vi "RevoxSerialTest.vi"() -> ()   [LabVIEW 2023]
uses:
  B203AllCluster.ctl
  B203Cluster.ctl
  <vilib>/Utility/error.llb/Trim Whitespace One-Sided.vi
  <instrlib>/_D2XX/D2XX/FT_Open_Device_By_Description.vi
  <instrlib>/_D2XX/D2XX-LV/private/FT_Status to Error.vi
  <instrlib>/_D2XX/D2XX-LV/API/Write Data (String).vi
  <instrlib>/_D2XX/D2XX-LV/API/Read Data (String).vi
  <instrlib>/_D2XX/D2XX-LV/D2XX-lv.lvlib
panel:
  out "String":string
  out "B203AllCluster":T1={"B203"={"Port"=enum."Anschluss 7", "Identifier"=0, "Language"=enum."Englisch", "Easy-Function"=enum."Easy Remote", "Timer-Function"=enum."Timer eingeschaltet", "Power ON condition"=enum."Lautsprecher A", "IR receiver"=enum."IR-Empfänger eingeschaltet"}, "Zeitstempel"=timestamp(0 s since 1904-01-01)} {"Zeitstempel" format="%<%x %.X>T"}
  in  "Stopp":bool
  in  "Schreibpuffer":string="0X"
  out "error out":errorcluster={"status"=FALSE, "code"=1073676294, "source"="VISA: Lesen in RevoxSerailTest.vi"} caption="Fehler (Ausgang)"
  in  "error in (no error)":errorcluster caption="Fehler (Eingang, kein Fehler)"
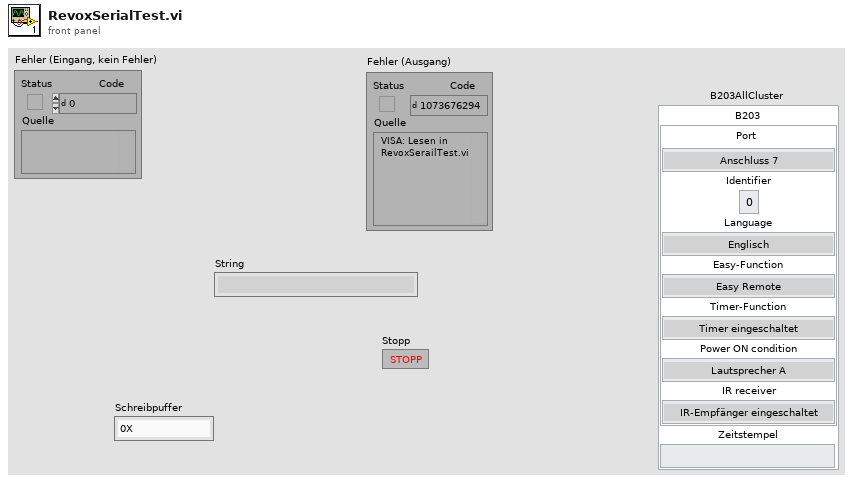
[diagram p1: front panel]
types:
  T1 = typedef "B203AllCluster.ctl" = cluster{"B203":T2, "Zeitstempel":timestamp}
  T2 = typedef "B203Cluster.ctl" = cluster{"Port":enum8{"B203-C", "Anschluss 1", "Anschluss 2", "Anschluss 3", "Anschluss 4", "Anschluss 5", "Anschluss 6", "Anschluss 7", "Anschluss 8", "Parallel Fernsteuerung"}, "Identifier":u8, "Language":enum8{"Englisch", "Deutsch", "Französich"}, "Easy-Function":enum8{"Easy Remote", "Easy Remote & Local", "Easy Off"}, "Timer-Function":enum8{"Timer eingeschaltet", "Timer ausgeschaltet"}, "Power ON condition":enum8{"Lautsprecher A", "Lautsprecher B", "Lautsprecher A & B", "Zuletzt aktivierte Lautespechergruppe", "Lautsprecher aus"}, "IR receiver":enum8{"IR-Empfänger eingeschaltet", "IR-Empfänger ausgeschaltet"}}
  T3 = cluster{"Word Length":u8, "Stop Bits":u8, "Parity":u8}
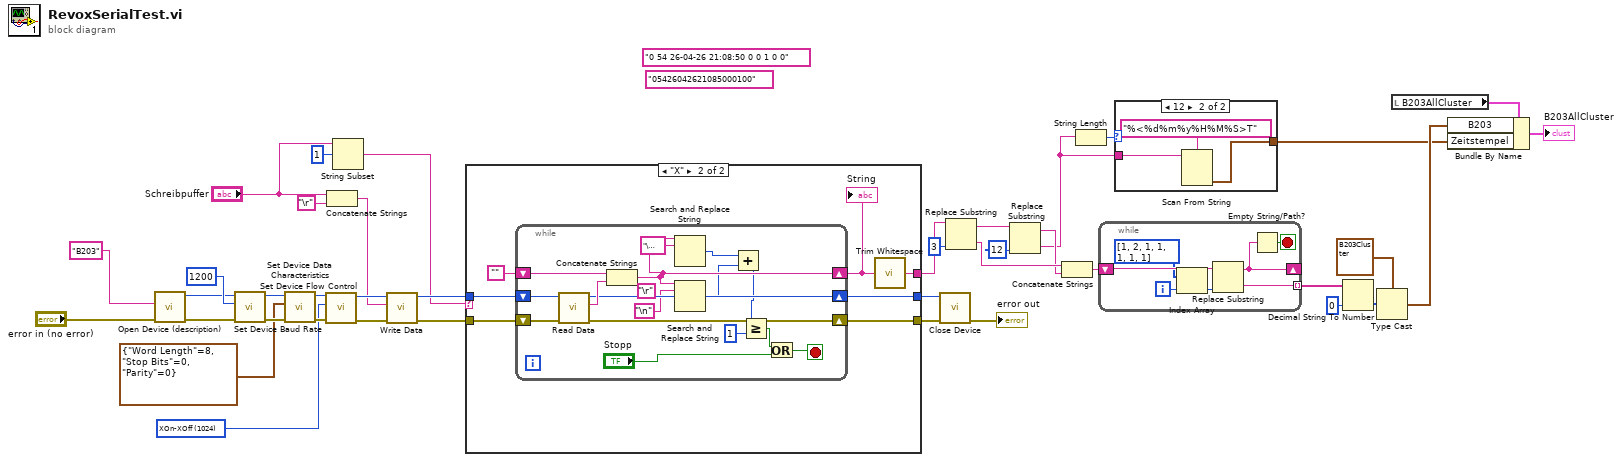
[diagram p0: block diagram]
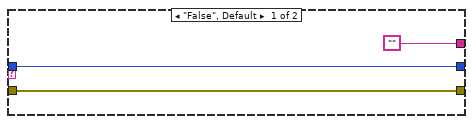
[diagram p2: hidden frame]
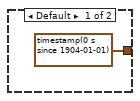
[diagram p3: hidden frame]
diagram:
  (unwired) "0 54 26-04-26 21:08:50 0 0 1 0 0"
  (unwired) "05426042621085000100"
  w34 = u16 1024 items=["None"=0, "RTS-CTS"=256, "DTR-DSR"=512, "XOn-XOff"=1024] ("Flow Control")
  n1 = call <instrlib>:"Open Device (description).vi"("error in (no error)"="error in (no error)", "Device Description"="B203") -> ("error out"=w24:errorcluster, "Handle"=w21:u64)  [unwired: 8 in]
  n2 = call <instrlib>:"Set Device Baud Rate.vi"("error in (no error)"=w24, "Baud Rate"=u32 1200 ("baud rate (9600)"), "Handle"=w21) -> ("error out"=w38:errorcluster, "Handle out"=w39:u64)  [unwired: 7 in]
  n3 = call <instrlib>:"Set Device Data Characteristics.vi"("error in (no error)"=w38, "Data Characteristics"=T3 {"Word Length"=8, "Stop Bits"=0, "Parity"=0}, "Handle"=w39) -> ("error out"=w35:errorcluster, "Handle out"=w33:u64)  [unwired: 7 in]
  n4 = call <instrlib>:"Set Device Flow Control.vi"("error in (no error)"=w35, "Flow Control"=w34, "Handle"=w33) -> ("error out"=w32:errorcluster, "Handle out"=w31:u64)  [unwired: 7 in]
  n5 = Concatenate Strings("Schreibpuffer", "\r") -> (w30:string)
  n6 = String Subset(string="Schreibpuffer", offset (0)=1 ("Offset (0)")) -> (substring=w2:string)  [unwired: 1 in]
  n7 = call-poly <instrlib>:"Write Data.vi"("error in (no error)"=w32, "Write Buffer"=w30, "Handle"=w31) -> ("error out"=w28:errorcluster, "Handle out"=w29:u64)  [unwired: 6 in, 1 out]
  n8 = case shown="\"X\"" w2 {
    tunnel: w29 -> [w43 w50]
    tunnel: w28 -> [w42 w49]
    tunnel: ["" w44] -> w1
    tunnel: [w42 w48] -> w27
    tunnel: [w43 w47] -> w26
    frame "False", Default {
    }
    frame "X" {
      n9 = while {
        shift-right: [w62] -> w47
        shift-left: w50 -> [w66]
        shift-right: [w63] -> w48
        shift-left: w49 -> [w65]
        shift-right: [w56] -> w45
        shift-left: "" -> [w61]
        stop <- w59 stop-if-true
        (unwired) "\r"
        n10 = call-poly <instrlib>:"Read Data.vi"("error in (no error)"=w65, "Handle"=w66) -> ("error out"=w63:errorcluster, "Read Buffer"=w64:string, "Handle out"=w62:u64)  [unwired: 6 in, 1 out]
        n11 = Concatenate Strings(w61, w64) -> (w56:string)
        n12 = Search and Replace String(input string=w56, search string="\u0007" ("Such-String")) -> (number of replacements=w54:i32)  [unwired: 6 in, 3 out]
        n13 = Search and Replace String(input string=w56, search string="\n") -> (number of replacements=w53:i32)  [unwired: 6 in, 3 out]
        n14 = Add(x=w54, y=w53) -> (x+y=w52:i32)
        n15 = Greater Or Equal?(x=w52, y=1) -> (x >= y?=w57:bool)
        n16 = Or(x=w57, y="Stopp") -> (x .or. y?=w59:bool)
      }
      "String" <- w45
      n17 = call <vilib>:"Trim Whitespace.vi"("string"=w45) -> ("trimmed string"=w44:string)  [unwired: 1 in]
    }
  }
  n18 = call <instrlib>:"Close Device.vi"("error in (no error)"=w27, "Handle"=w26) -> ("error out"=→"error out":errorcluster)  [unwired: 9 in]
  n19 = Replace Substring(2:3 ("Länge (Länge des Teil-Strings)"), 5:w1) -> (0:w14:string, 1:w16:string)  [unwired: 2 in]
  n20 = Replace Substring(2:12 ("Länge (Länge des Teil-Strings)"), 5:w16) -> (0:w10:string, 1:w13:string)  [unwired: 2 in]
  n21 = Concatenate Strings(w14, w13) -> (w12:string)
  n22 = String Length(string=w10) -> (length=w11:i32)
  n23 = while {
    shift-right: [w71] -> _
    shift-left: w12 -> [w73]
    tunnel: [w70] -> w20 mode=indexing
    i -> [w69]
    stop <- w72 stop-if-true
    n24 = Index Array(array=i32[] [1, 2, 1, 1, 1, 1, 1], index=w69) -> (element=w68:i32)
    n25 = Replace Substring(2:w68, 5:w73) -> (0:w70:string, 1:w71:string)  [unwired: 2 in]
    n26 = Empty String/Path?(string/path=w71) -> (empty?=w72:bool)
  }
  n27 = case shown="12" w11 {
    tunnel: w10 -> [_ w77]
    tunnel: [timestamp(0 s since 1904-01-01) w75] -> w6
    frame Default {
    }
    frame 12 {
      n28 = Scan From String(format string="%<%d%m%y%H%M%S>T" ("Format-String"), input string=w77) -> (output 1=w75:timestamp)  [unwired: 3 in, 3 out]
    }
  }
  n29 = Decimal String To Number(string=w20, default (0L)=u8 0 ("Standard (0 I32)")) -> (number=w18:u8[])  [unwired: 1 in, 1 out]
  n30 = Type Cast(type=T2 {"Port"=enum."B203-C", "Identifier"=54, "Language"=enum."Englisch", "Easy-Function"=enum."Easy Remote", "Timer-Function"=enum."Timer eingeschaltet", "Power ON condition"=enum."Lautsprecher A", "IR receiver"=enum."IR-Empfänger eingeschaltet"} ("Wert"), x=w18) -> (*(type *) &x=w7:T2)
  n31 = local read "B203AllCluster"() -> (w9:T1)
  n32 = Bundle By Name(cluster=w9, "B203"=w7, "Zeitstempel"=w6) -> (→"B203AllCluster":T1)
